vi "MenuHandler.vi"(5 "tree control":refnum<vi>, 7 "main queue":refnum<queue>, 8 "error in":errorcluster, 9 "parameters":variant, 10 "menu string":string, 11 "ACIR Instrument":refnum<class "ACIR Instrument.lvclass">) -> (0 "error out":errorcluster, 1 "refresh tree?":bool, 2 "Unhandled":bool, 3 "ACIR Instrument out":refnum<class "ACIR Instrument.lvclass">)   [LabVIEW 2025, in "ACIR.lvlib" / "ACIR Instrument.lvclass"]
doc: "Copyright 2017 National Instruments Corporation\n\nLicensed under the Apache License, Version 2.0 (the \"License\"); you may not use this file except in compliance with the License. You may obtain a copy of the License at http://www.apache.org/licenses/LICENSE-2.0\nUnless required by applicable law or agreed to in writing, software distributed under the License is distributed on an \"AS IS\" BASIS, WITHOUT WARRANTIES OR CONDITIONS OF ANY KIND, either express or implied. See the License for the specific language governing permissions and limitations under the License."
uses:
  ACIR Instrument.lvclass
  Users/Public/Documents/Sandia National Labs/TSS Plugin/Abstract Engine.lvlibp/Abstract Instrument/Abstract Instrument.lvclass
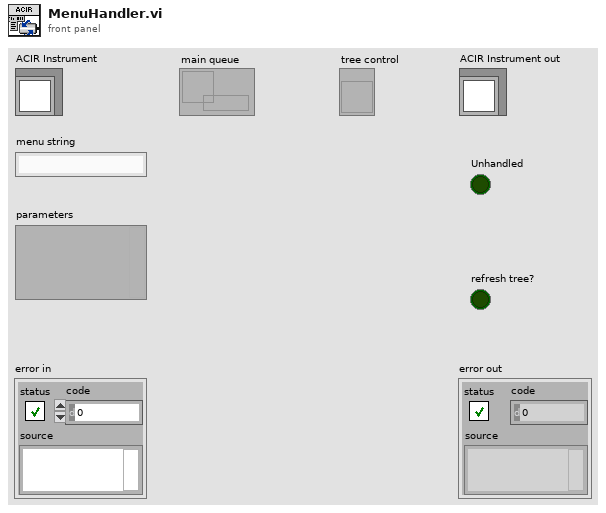
[diagram p1: front panel]
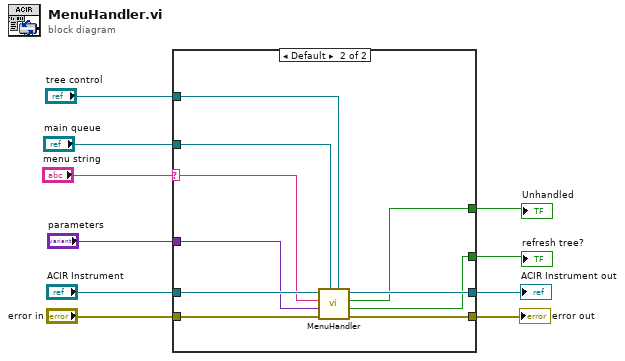
[diagram p0: block diagram]
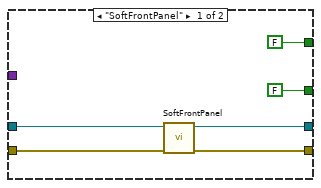
[diagram p2: hidden frame]
diagram:
  n1 = case shown="Default" "menu string" {
    selector: "menu string" -> [_ w20]
    tunnel: "error in" -> [w12 w26]
    tunnel: [w11 w25] -> w8
    tunnel: "ACIR Instrument" -> [w14 w24]
    tunnel: [w13 w23] -> w6
    tunnel: [FALSE ("refresh tree?") w21] -> w5
    tunnel: [FALSE ("Unhandled") w22] -> w4
    tunnel: "main queue" -> [_ w19]
    tunnel: "tree control" -> [_ w18]
    tunnel: "parameters" -> [_ w17]
    frame "SoftFrontPanel" {
      n2 = call "SoftFrontPanel.vi"("error in (no error)"=w12, "ACIR Instrument"=w14) -> ("error out"=w11:errorcluster, "ACIR Instrument out"=w13:refnum<class "ACIR Instrument.lvclass">)  [unwired: 8 in]
    }
    frame Default {
      n3 = call-parent "MenuHandler.vi"("tree control"=w18, "main queue"=w19, "error in"=w26, "parameters"=w17, "menu string"=w20, "CEF_serializable node in"=w24) -> ("error out"=w25:errorcluster, "refresh tree?"=w21:bool, "Unhandled"=w22:bool, "CEF_serializable node out"=w23:refnum<class "ACIR Instrument.lvclass">)  [unwired: 2 in]
    }
  }
  "error out" <- w8
  "ACIR Instrument out" <- w6
  "Unhandled" <- w4
  "refresh tree?" <- w5
